vi "NewControl258297343.vi"(6 "timeout in ms (-1)":i32=-1, 8 "error in (no error)":errorcluster, 9 "asdf":dbl, 10 "String":string, 11 "module in":refnum<class "TemplateModule.lvclass">) -> (0 "error out":errorcluster, 1 "asdf 2":dbl, 2 "String 2":string, 3 "module out":refnum<class "TemplateModule.lvclass">, 4 "timed out?":bool)   [LabVIEW 2024]
uses:
  TemplateModule.lvclass/TemplateModule.ctl
  JQMHCore/Module/JQMHModule.lvclass
  JQMHCore/Module/Reply.ctl
  NewControl258297343 Args.ctl
  NewControl258297343 ReplyArgs.ctl
  TemplateModule.lvclass
  C:/Github/JQMH/JQMHCore/Module/JQMHModule.lvclass
  C:/Github/JQMH/Scripting/templates/TemplateModule/TemplateModule.lvclass
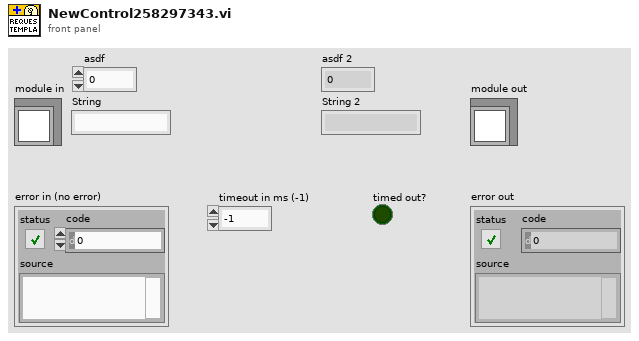
[diagram p1: front panel]
types:
  T1 = typedef "NewControl258297343 Args.ctl" = cluster{"asdf":dbl, "String":string}
  T2 = typedef "JQMHModule.lvclass/Reply.ctl" = cluster{"Expects Reply":bool, "Reply":refnum<notifier>}
  T3 = typedef "NewControl258297343 ReplyArgs.ctl" = cluster{"asdf":dbl, "String":string}
  T4 = cluster{"RQMH_REPLYARGS":T3, "error in (no error)":errorcluster}
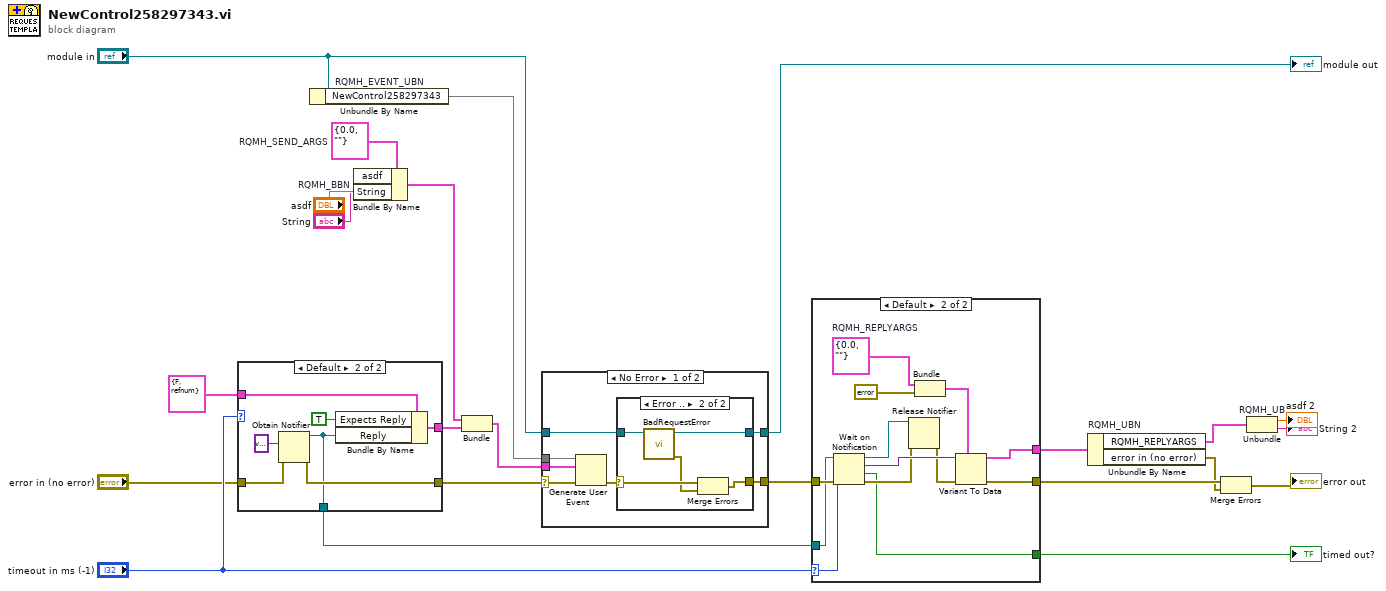
[diagram p0: block diagram]
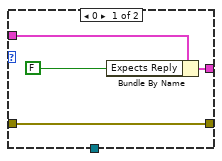
[diagram p4: hidden frame]
diagram:
  w13 = T1 {"asdf"=0.0, "String"=""}  # RQMH_SEND_ARGS
  n1 = case shown="Default" "timeout in ms (-1)" {
    tunnel: [w26 w33] -> w23
    tunnel: "error in (no error)" -> [w24 w32]
    tunnel: [w24 w31] -> w21
    tunnel: [_ w30] -> w19
    tunnel: T2 {"Expects Reply"=FALSE, "Reply"=refnum} ("Reply") -> [w27 w29]
    frame 0 {
      n2 = Bundle By Name(cluster=w27, "Expects Reply"=FALSE) -> (w26:T2)
    }
    frame Default {
      n3 = Obtain Notifier(notification data type=variant, error in (no error)=w32) -> (notifier out=w30:refnum<notifier>, error out=w31:errorcluster)  [unwired: 2 in, 1 out]
      n4 = Bundle By Name(cluster=w29, "Expects Reply"=TRUE, "Reply"=w30) -> (w33:T2)
    }
  }
  n5 = Unbundle By Name "RQMH_EVENT_UBN"("module in") -> ("NewControl258297343"=w11)
  n6 = Bundle By Name "RQMH_BBN"(cluster=w13, "asdf"="asdf", "String"="String") -> (w10:T1)
  n7 = Bundle("RQMH_SEND_ARGS"=w10, "Reply"=w23) -> (w22:cluster{"RQMH_SEND_ARGS":T1, "Reply":T2})  [unwired: 1 in]
  n8 = case shown="No Error" w21 {
    selector: w21 -> [w38 w49]
    tunnel: w22 -> [w41 _]
    tunnel: w11 -> [w40 _]
    tunnel: [w37 w49] -> w20
    tunnel: "module in" -> [w36 w50]
    tunnel: [w35 w50] -> w14
    frame No Error {
      n9 = Generate User Event(user event=w40, event data cluster=w41, error in=w38) -> (error out=w39:errorcluster)  [unwired: 1 in, 1 out]
      n10 = case shown="Error .." w39 {
        selector: w39 -> [w42 w48]
        tunnel: [w42 w47] -> w37
        tunnel: w36 -> [w43 w46]
        tunnel: [w43 w45] -> w35
        frame No Error {
        }
        frame Error {
          n11 = call "BadRequestError.vi"("JQMHModule in"=w46) -> ("error out"=w44:errorcluster, "JQMHModule out"=w45:refnum<class "TemplateModule.lvclass">)  [unwired: 9 in]
          n12 = Merge Errors(w48, w44) -> (w47:errorcluster)
        }
      }
    }
    frame Error {
    }
  }
  "module out" <- w14
  n13 = case shown="Default" "timeout in ms (-1)" {
    selector: "timeout in ms (-1)" -> [_ w55]
    tunnel: w20 -> [w51 w64]
    tunnel: w19 -> [_ w63]
    tunnel: [_ w56] -> w18
    tunnel: [w51 w53] -> w9
    tunnel: [_ w52] -> w8
    frame 0 {
    }
    frame Default {
      w54 = T3 {"asdf"=0.0, "String"=""}  # RQMH_REPLYARGS
      n14 = Wait on Notification(notifier=w63, timeout in ms (-1)=w55, error in (no error)=w64) -> (notifier out=w59:refnum<notifier>, notification=w60:variant, timed out?=w56:bool, error out=w58:errorcluster)  [unwired: 1 in]
      n15 = Release Notifier(notifier=w59, error in (no error)=w58) -> (error out=w57:errorcluster)  [unwired: 1 in, 2 out]
      n16 = Bundle("RQMH_REPLYARGS"=w54, "error in (no error)"=errorcluster {"status"=FALSE, "code"=0, "source"=""}) -> (w62:T4)  [unwired: 1 in]
      n17 = Variant To Data(error in=w57, type=w62, Variant=w60) -> (data=w52:T4, error out=w53:errorcluster)
    }
  }
  "timed out?" <- w18
  n18 = Unbundle By Name "RQMH_UBN"(w8) -> ("RQMH_REPLYARGS"=w5:T3, "error in (no error)"=w6:errorcluster)
  n19 = Merge Errors(w9, w6) -> (→"error out":errorcluster)
  n20 = Unbundle "RQMH_UB"(w5) -> ("asdf"=→"asdf 2":dbl, "String"=→"String 2":string)
